vi "MB Ethernet Slave Demon - Single Port - Multiple Connections.vi"(9 "Period":u32=200, 10 "Timeout":i32=5000, 11 "Port":u16=502) -> (2 "Demon Running":bool, 3 "# of connections":i32)   [LabVIEW 2011]
uses:
  MB Ethernet Connection Function.ctl
  <vilib>/Platform/TimedLoop/XDataNode/timing_clust.ctl
  <vilib>/Platform/TimedLoop/XDataNode/nitl_modes.ctl
  <vilib>/Platform/TimedLoop/XDataNode/wakeup.ctl
  MB Globals.vi
  <vilib>/Platform/TimedLoop/XDataNode/XDataNode.xnode
  <vilib>/Platform/TimedLoop/XDataNode/XDNodeRunTimeDep.lvlib
panel:
  # "VI Name: MB Ethernet Slave Demon.vi\nPurpose: Modbus Demon\nMonitor a single port, but can accept multiple connections."
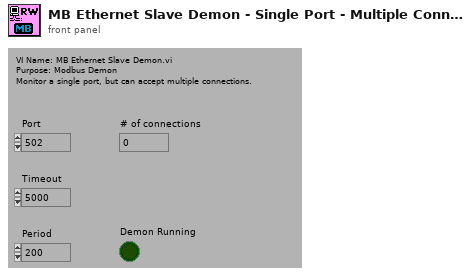
[diagram p1: front panel]
types:
  T1 = typedef "MB Ethernet Connection Function.ctl" = enum16{"Init", "Add Connection", "Get All Connections", "Delete Connection"}
  T2 = typedef "XDNodeRunTimeDep.lvlib/timing_clust.ctl" = cluster{"Expected End [f-1]":u64, "Actual End [f-1]":u64, "Finished Late? [f-1]":bool, "Expected End [i-1]":u64, "Actual End [i-1]":u64, "Finished Late? [i-1]":bool, "Expected Start [i]":u64, "Actual Start [i]":u64, "Expected Start [f]":u64, "Actual Start [f]":u64, "Source Name":string, "Structure Name":string, "Period":i64, "Deadline":i64, "Offset":i64, "Start":i64, "Priority":i32, "Timeout":i32, "Mode":T3, "Wakeup Reason":T4, "Error":errorcluster, "Source Type":string, "Secondary Source Type":string, "Global End Time":u64, "Global Start Time":u64, "Frame Duration":u64, "Iteration Duration":u64, "Assigned CPU":i32, "I/O Scan Engine Mode":u32}
  T3 = typedef "XDNodeRunTimeDep.lvlib/nitl_modes.ctl" = enum32{"No Change", "Process missed periods, maintain original phase", "Discard missed periods, maintain original phase", "Process missed periods, ignore original phase", "Discard missed periods, ignore original phase"}
  T4 = typedef "XDNodeRunTimeDep.lvlib/wakeup.ctl" = enum32{"Normal", "Aborted", "Asynchronous wakeup", "Timing source error", "Timed loop error", "Timeout"}
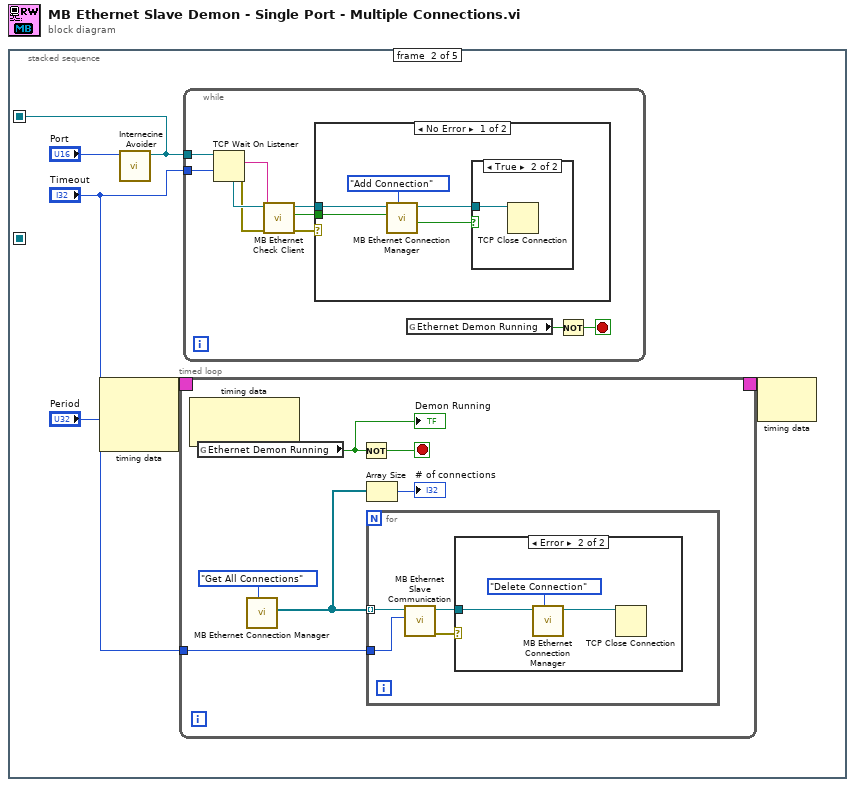
[diagram p0: block diagram]
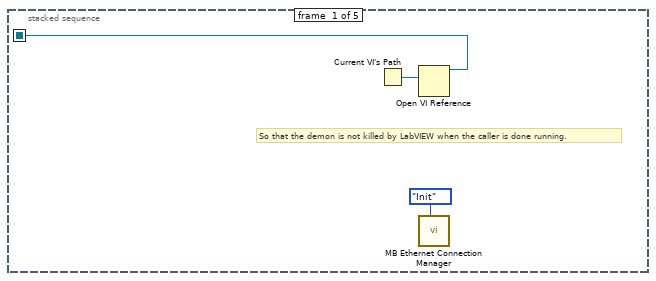
[diagram p2: hidden frame]
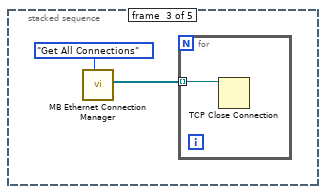
[diagram p6: hidden frame]
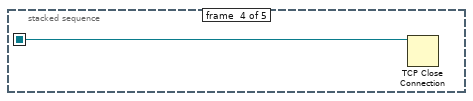
[diagram p7: hidden frame]
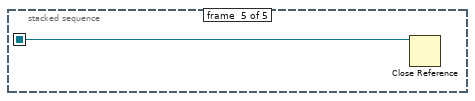
[diagram p8: hidden frame]
diagram:
  n1 = stacked-sequence {
    seq-local: [w2 _ _ _ _] -> [_ _ _ _ w49]
    seq-local: [_ w6 _ _ _] -> [_ _ _ w48 _]
    frame #0 {
      # "So that the demon is not killed by LabVIEW when the caller is done running."
      n2 = Current VI's Path() -> (path=w3:path)
      n3 = Open VI Reference(vi path=w3) -> (vi reference=w2:refnum<vi>)  [unwired: 1 in, 5 out]
      n4 = call "MB Ethernet Connection Manager.vi"("Function"=MB_Ethernet_Connection_Function."Init") -> ()  [unwired: 2 in, 9 out]
    }
    frame #1 {
      n5 = node-c288("Period") -> (w4:T2)  [unwired: 2 out]
      n6 = call <vilib>:"Internecine Avoider.vi"("port"="Port") -> ("connection ID"=w6:refnum<k5>)  [unwired: 3 in, 7 out]
      n7 = timed-loop {
        tunnel: "Timeout" -> [w13]
        timing-out: [_] -> w5
        timing: w4 -> [_]
        stop <- w15 stop-if-true
        n8 = node-c288() -> ()  [unwired: 3 out]
        n9 = global read "MB Globals.vi" "Ethernet Demon Running"() -> (w14:bool)
        "Demon Running" <- w14
        n10 = call "MB Ethernet Connection Manager.vi"("Function"=MB_Ethernet_Connection_Function."Get All Connections") -> ("Connection IDs"=w11:refnum<k5>[])  [unwired: 2 in, 8 out]
        n11 = Not(x=w14) -> (.not. x?=w15:bool)
        n12 = Array Size(array=w11) -> (size(s)=→"# of connections":i32)
        n13 = for {
          tunnel: w13 -> [w19]
          tunnel: w11 -> [w17] mode=indexing
          n14 = call "MB Ethernet Slave Communication.vi"("Timeout"=w19, "Connection ID"=w17) -> ("error out"=w20:errorcluster, "Connection ID (dup)"=w18:refnum<k5>)  [unwired: 1 in, 7 out]
          n15 = case shown="Error" w20 {
            tunnel: w18 -> [_ w22]
            frame No Error {
            }
            frame Error {
              n16 = call "MB Ethernet Connection Manager.vi"("Function"=MB_Ethernet_Connection_Function."Delete Connection", "Connection ID"=w22) -> ("Connection ID to Delete"=w21:refnum<k5>)  [unwired: 1 in, 8 out]
              n17 = TCP Close Connection(connection ID=w21) -> ()  [unwired: 1 in, 3 out]
            }
          }
        }
      }
      n18 = while {
        tunnel: w6 -> [w38]
        tunnel: "Timeout" -> [w35]
        stop <- w36 stop-if-true
        n19 = TCP Wait On Listener(9:w35, 11:w38) -> (0:w32:errorcluster, 2:w30:string, 4:w34:refnum<k5>)  [unwired: 1 in, 3 out]
        n20 = call "MB Ethernet Check Client.vi"("error in (no error)"=w32, "Remote Address"=w30, "Connection ID in"=w34) -> ("error out"=w31:errorcluster, "Priority"=w29:bool, "Connection ID out"=w33:refnum<k5>)  [unwired: 6 out]
        n21 = case shown="No Error" w31 {
          tunnel: w33 -> [w43 _]
          tunnel: w29 -> [w39 _]
          frame No Error {
            n22 = call "MB Ethernet Connection Manager.vi"("Function"=MB_Ethernet_Connection_Function."Add Connection", "Priority"=w39, "Connection ID"=w43) -> ("Close Connection"=w41:bool, "Connection ID to Delete"=w40:refnum<k5>)  [unwired: 7 out]
            n23 = case shown="True" w41 {
              tunnel: w40 -> [_ w44]
              frame False {
              }
              frame True {
                n24 = TCP Close Connection(connection ID=w44) -> ()  [unwired: 1 in, 3 out]
              }
            }
          }
          frame Error {
          }
        }
        n25 = global read "MB Globals.vi" "Ethernet Demon Running"() -> (w37:bool)
        n26 = Not(x=w37) -> (.not. x?=w36:bool)
      }
      n27 = node-c288(w5) -> ()  [unwired: 1 out]
    }
    frame #2 {
      n28 = call "MB Ethernet Connection Manager.vi"("Function"=MB_Ethernet_Connection_Function."Get All Connections") -> ("Connection IDs"=w45:refnum<k5>[])  [unwired: 2 in, 8 out]
      n29 = for {
        tunnel: w45 -> [w47] mode=indexing
        n30 = TCP Close Connection(connection ID=w47) -> ()  [unwired: 1 in, 3 out]
      }
    }
    frame #3 {
      n31 = TCP Close Connection(connection ID=w48) -> ()  [unwired: 1 in, 3 out]
    }
    frame #4 {
      n32 = Close Reference(reference=w49) -> ()  [unwired: 1 in, 1 out]
    }
  }
